vi "Calculate point-averaged current.vi"(10 "No. of data point averages":i32, 11 "Current list":sgl[](array[numeric])) -> (3 "Point-averaged current":sgl[](array[numeric]))   [LabVIEW 2011]
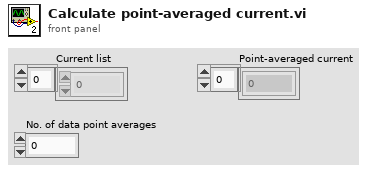
[diagram p1: front panel]
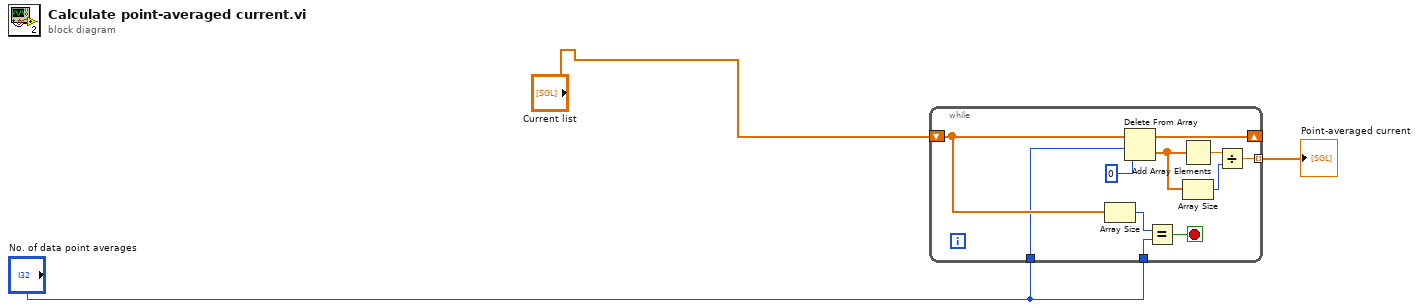
[diagram p0: block diagram]
diagram:
  n1 = while {
    shift-right: [w10] -> _
    shift-left: "Current list" -> [w12]
    tunnel: [w6] -> w2 mode=indexing
    tunnel: "No. of data point averages" -> [w5]
    tunnel: "No. of data point averages" -> [w4]
    stop <- w13 stop-if-true
    n2 = Array Size(array=w12) -> (size(s)=w14:i32)
    n3 = Delete From Array(array=w12, length=w4, index=0) -> (deleted portion=w8:sgl[], array with subset deleted=w10:sgl[])
    n4 = Equal?(x=w14, y=w5) -> (x = y?=w13:bool)
    n5 = Add Array Elements(numeric array=w8) -> (sum=w9:sgl)
    n6 = Array Size(array=w8) -> (size(s)=w7:i32)
    n7 = Divide(x=w9, y=w7) -> (x/y=w6:sgl)
  }
  "Point-averaged current" <- w2
